vi "Init Events.vi"(8 "Error In":errorcluster, 11 "WebView in":refnum<class "WebView.lvclass">) -> (0 "Error Out":errorcluster, 3 "WebView out":refnum<class "WebView.lvclass">)   [LabVIEW 2024, in "WebView.lvclass"]
uses:
  WebView.lvclass
  Source Changed Event Data--cluster.ctl
  Events--cluster.ctl
  Navigation Complete Event Data--cluster.ctl
  Navigation Start Event Data--cluster.ctl
  WebView.lvclass/WebView.ctl
  <vilib>/sklein/WebView2/Libs/Microsoft.Web.WebView2.Core.dll
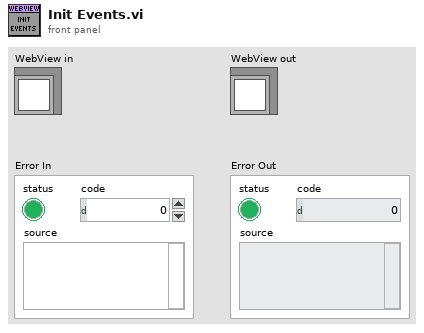
[diagram p1: front panel]
types:
  T1 = typedef "WebView.lvclass/Navigation Start Event Data--cluster.ctl" = cluster{"AdditionalAllowedFrameAncestors":string, "Cancel":bool, "IsRedirected":bool, "IsUserInitiated":bool, "NavigationId":u64, "NavigationKind":i32, "RequestHeaders":refnum<k24>, "Uri":string}
  T2 = typedef "WebView.lvclass/Navigation Complete Event Data--cluster.ctl" = cluster{"HttpStatusCode":i32, "IsSuccess?":bool, "NavigationId":u64, "WebErrorStatus":i32}
  T3 = cluster{"Source":string, "WebMessageAsJson":string}
  T4 = typedef "WebView.lvclass/Events--cluster.ctl" = cluster{"Navigation Complete Event":refnum<user-event>, "Source Changed Event":refnum<user-event>, "Document Title Changed Event":refnum<user-event>, "Status Bar Text Changed":refnum<user-event>, "Web Message Received":refnum<user-event>, "Window Close Requested":refnum<user-event>, "DOM Loaded":refnum<user-event>, "Navigation Started Event":refnum<user-event>}
  T5 = typedef "WebView.lvclass/Source Changed Event Data--cluster.ctl" = cluster{"Source":string, "IsNewDocument":bool}
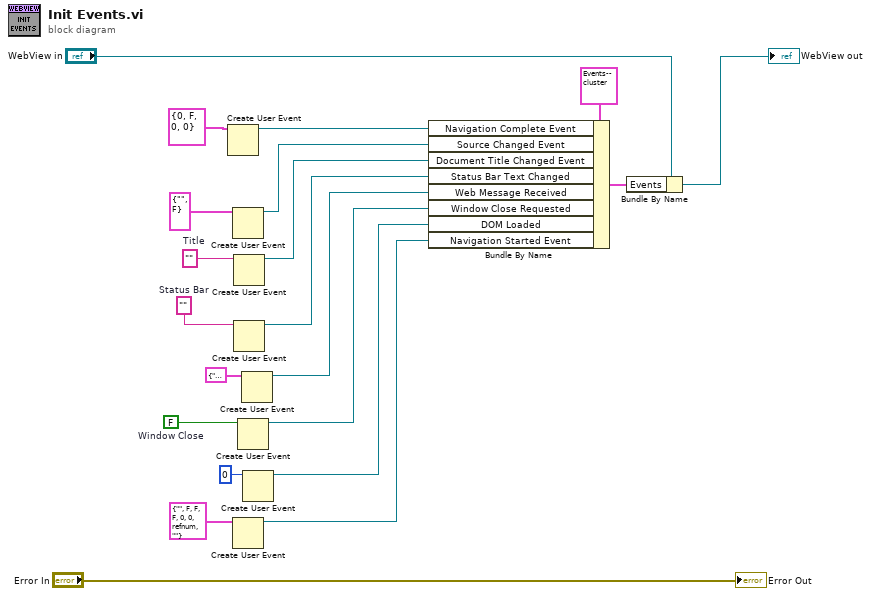
[diagram p0: block diagram]
diagram:
  w12 = FALSE  # Window Close
  w9 = ""  # Status Bar
  w4 = ""  # Title
  n1 = Create User Event(user event datatype=T2 {"HttpStatusCode"=0, "IsSuccess?"=FALSE, "NavigationId"=0, "WebErrorStatus"=0} ("output cluster")) -> (user event=w7:refnum<user-event>)  [unwired: 1 in, 1 out]
  n2 = Create User Event(user event datatype=T5 {"Source"="", "IsNewDocument"=FALSE} ("Source")) -> (user event=w8:refnum<user-event>)  [unwired: 1 in, 1 out]
  n3 = Create User Event(user event datatype=T1 {"AdditionalAllowedFrameAncestors"="", "Cancel"=FALSE, "IsRedirected"=FALSE, "IsUserInitiated"=FALSE, "NavigationId"=0, "NavigationKind"=0, "RequestHeaders"=refnum, "Uri"=""} ("Nav Started Event")) -> (user event=w18:refnum<user-event>)  [unwired: 1 in, 1 out]
  n4 = Create User Event(user event datatype=w4) -> (user event=w6:refnum<user-event>)  [unwired: 1 in, 1 out]
  n5 = Create User Event(user event datatype=w9) -> (user event=w10:refnum<user-event>)  [unwired: 1 in, 1 out]
  n6 = Create User Event(user event datatype=w12) -> (user event=w13:refnum<user-event>)  [unwired: 1 in, 1 out]
  n7 = Create User Event(user event datatype=T3 {"Source"="", "WebMessageAsJson"=""} ("output cluster")) -> (user event=w11:refnum<user-event>)  [unwired: 1 in, 1 out]
  n8 = Create User Event(user event datatype=u64 0 ("NavigationId")) -> (user event=w15:refnum<user-event>)  [unwired: 1 in, 1 out]
  n9 = Bundle By Name(cluster=T4 {"Navigation Complete Event"=refnum, "Source Changed Event"=refnum, "Document Title Changed Event"=refnum, "Status Bar Text Changed"=refnum, "Web Message Received"=refnum, "Window Close Requested"=refnum, "DOM Loaded"=refnum, "Navigation Started Event"=refnum} ("Cluster"), "Navigation Complete Event"=w7, "Source Changed Event"=w8, "Document Title Changed Event"=w6, "Status Bar Text Changed"=w10, "Web Message Received"=w11, "Window Close Requested"=w13, "DOM Loaded"=w15, "Navigation Started Event"=w18) -> (w20:T4)
  n10 = Bundle By Name(cluster="WebView in", "Events"=w20) -> (→"WebView out":refnum<class "WebView.lvclass">)
  "Error Out" <- "Error In"
